vi "ReadData_9234.vi"(8 "error in":errorcluster, 11 "Module Config Selector":i16) -> (0 "error out":errorcluster, 3 "Data Array":sgl[](array[numeric]) format="%.2f")   [LabVIEW 2017, in "BOP_VibAPI_2.lvlib"]
uses:
  <vilib>/addons/InsightCM/Devices/Shared/Cms/Fpga/Acquisition/source/subVIs/VibAPI_2/BOP_VibAPI_2.lvlib
  <vilib>/rvi/eio/common/nirviEmuTemplateMethod_errors.vi
  <vilib>/eio/EIONode/EIONode.xnode
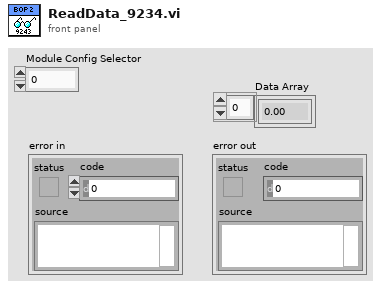
[diagram p1: front panel]
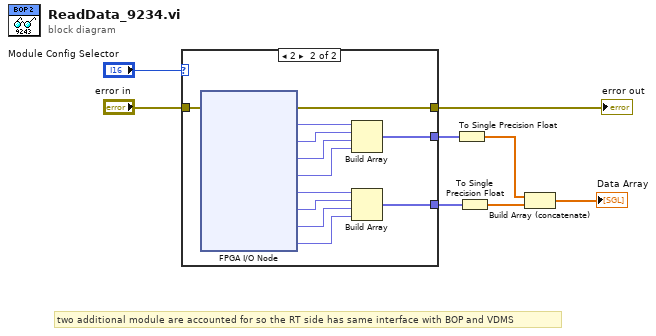
[diagram p0: block diagram]
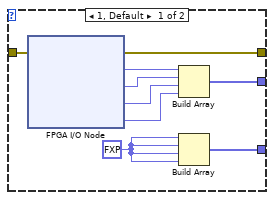
[diagram p2: hidden frame]
diagram:
  # "two additional module are accounted for so the RT side has same interface with BOP and VDMS"
  n1 = case shown="2" "Module Config Selector" {
    tunnel: "error in" -> [w14 w26]
    tunnel: [w13 w25] -> w7
    tunnel: [w11 w24] -> w4
    tunnel: [w12 w23] -> w2
    frame 1, Default {
      w9 = fxp<+/-,24,7> 0.0 ("Mod1/AI2")
      n2 = xnode "FPGA I/O Node"("error in"=w14) -> ("error out"=w13:errorcluster, "Mod1/AI0"=w15:fxp<+/-,24,4>, "Mod1/AI1"=w17:fxp<+/-,24,4>, "Mod1/AI2"=w16:fxp<+/-,24,4>, "Mod1/AI3"=w10:fxp<+/-,24,4>)  [unwired: 4 in, 4 out]
      n3 = Build Array(w15, w17, w16, w10) -> (w11:fxp<+/-,24,4>[])
      n4 = Build Array(w9, w9, w9, w9) -> (w12:fxp<+/-,24,7>[])
    }
    frame 2 {
      n5 = xnode "FPGA I/O Node"("error in"=w26) -> ("error out"=w25:errorcluster, "Mod1/AI0"=w27:fxp<+/-,24,4>, "Mod1/AI1"=w29:fxp<+/-,24,4>, "Mod1/AI2"=w28:fxp<+/-,24,4>, "Mod1/AI3"=w22:fxp<+/-,24,4>, "Mod2/AI0"=w21:fxp<+/-,24,4>, "Mod2/AI1"=w20:fxp<+/-,24,4>, "Mod2/AI2"=w19:fxp<+/-,24,4>, "Mod2/AI3"=w18:fxp<+/-,24,4>)  [unwired: 8 in, 8 out]
      n6 = Build Array(w27, w29, w28, w22) -> (w24:fxp<+/-,24,4>[])
      n7 = Build Array(w21, w20, w19, w18) -> (w23:fxp<+/-,24,4>[])
    }
  }
  "error out" <- w7
  n8 = To Single Precision Float(number=w4) -> (single precision float=w3:sgl[])
  n9 = To Single Precision Float(number=w2) -> (single precision float=w1:sgl[])
  n10 = Build Array (concatenate)(w3, w1) -> (→"Data Array":sgl[])
